vi "UHR-Fleezers Control (host) - 10.8.vi"() -> ()   [LabVIEW 2013] (continued)
        n493 = local write "Load parameters"(FALSE ("Load parameters")) -> ()
        n494 = Index Array(array="Saved AOD Raster Scan Parameter Sets", index=w859) -> (element=w858:T32)
        n495 = Unbundle By Name(w858) -> ("Scan Range AOD (nm) 2"=w857:dbl, "Step Size AOD (nm) 2"=w856:dbl, "Scan Speed AOD (nm/s) 2"=w855:dbl, "Number of scans (AOD) 2"=w854:u16)
        n496 = flat-sequence {
          tunnel: w857 -> [w865]
          tunnel: w856 -> [w864]
          tunnel: w855 -> [w863]
          tunnel: w854 -> [w866]
          frame #0 {
            n497 = local write "Scan Speed (nm/s)"(w863) -> ()
            n498 = local write "Scan Range (nm)"(w865) -> ()
            n499 = local write "Step Size (nm)"(w864) -> ()
          }
          frame #1 {
            n500 = property on="Number of F/B Scans (AOD)" class="DigNum (strict)"("Val(Sgnl)"=w866) -> ()  [unwired: 2 in, 2 out]
          }
        }
      }
      event "Trap 1 (ON/OFF)", "Trap 2 (ON/OFF)": Value Change {
        n501 = event-data() -> ()  [unwired: 7 out]
        n502 = property on="Trap 2 ON" class="Bool (strict)"("Val(Sgnl)"="Trap 2 (ON/OFF)") -> ()  [unwired: 2 in, 2 out]
        n503 = property on="Trap 1 ON" class="Bool (strict)"("Val(Sgnl)"="Trap 1 (ON/OFF)") -> ()  [unwired: 2 in, 2 out]
      }
      event "DIO count 1 (ticks)", "DIO count 2 (ticks)", "DIO count 3 (ticks)", "Interlace", "Number Interlace Sets", "Not-Interlacing Set": Value Change {
        n504 = event-data() -> ()  [unwired: 7 out]
        n505 = local read "DIO count 3 (ticks)"() -> (w879:u32)
        n506 = local read "DIO count 1 (ticks)"() -> (w881:u32)
        n507 = local read "DIO count 2 (ticks)"() -> (w880:u32)
        n508 = To Unsigned Byte Integer(number="Not-Interlacing Set") -> (unsigned 8bit integer=w870:u8)
        n509 = Add(x=w870, y=u8 1) -> (x+y=w874:u8)
        n510 = xnode "Read/Write Control"("FPGA VI Reference In"=w885, "error in"=w883, "DIO count 1 (ticks)"=w881, "DIO count 2 (ticks)"=w880, "DIO count 3 (ticks)"=w879, "Interlace ON/OFF"="Interlace", "Number Interlace Cycles"="Number Interlace Sets", "Interlace Off Parameters"=w874) -> ("error out"=w884:errorcluster)  [unwired: 1 out]
        n511 = Build Array(w881, w880, w879) -> (w872:u32[])
        n512 = Split 1D Array(array=w872, index="Number Interlace Sets") -> (first subarray=w882:u32[])  [unwired: 1 out]
        n513 = Index Array(array=w872, index=w870) -> (element=w871:u32)
        n514 = Add Array Elements(numeric array=w882) -> (sum=w876:u32)
        n515 = Select(t=w876, s="Interlace", f=w871) -> (s? t:f=→"Total Counts (ticks)":u32)
      }
      event "Reset Feedback": Value Change {
        n516 = event-data() -> ()  [unwired: 7 out]
        n517 = Unbundle By Name("Reset Feedback") -> ("Set 1"=w889:bool, "Set 2"=w888:bool)
        n518 = xnode "Read/Write Control"("FPGA VI Reference In"=w891, "error in"=w886, "FB Reset Set 1"=w889, "FB Reset Set 2"=w888) -> ("error out"=w887:errorcluster)  [unwired: 1 out]
      }
      event "PID Gains": Value Change {
        n519 = event-data() -> ()  [unwired: 7 out]
        n520 = Unbundle By Name("PID Gains") -> ("Set 1"=w895:T14, "Set 2"=w894:T14)
        n521 = xnode "Read/Write Control"("FPGA VI Reference In"=w896, "error in"=w892, "FB Gains Set 1"=w895, "FB Gains Set 2"=w894) -> ("error out"=w893:errorcluster)  [unwired: 1 out]
      }
      event "AI2 to Setpoint", "Trap Intensity\nSetpoints (V)": Value Change {
        n522 = event-data() -> ()  [unwired: 7 out]
        n523 = xnode "Read/Write Control"("FPGA VI Reference In"=w902, "error in"=w898) -> ("FPGA VI Reference Out"=w901:T19, "error out"=w900:errorcluster, "AI2 Y Sum Set 1"=w909:i16, "AI2 Y Sum Set 2"=w908:i16)
        n524 = Cluster To Array(cluster="AI2 to Setpoint") -> (array=w912:bool[])
        n525 = local read "AI2 (V)"() -> (w910:cluster{"Set 1":dbl, "Set 2":dbl})
        n526 = Or Array Elements(Boolean array=w912) -> (logical OR=w913:bool)
        n527 = Bundle By Name(cluster=w910, "Set 1"=w909, "Set 2"=w908) -> (w907:cluster{"Set 1":dbl, "Set 2":dbl})
        n528 = Divide(x=w907, y=3276.7) -> (x/y=w906:cluster{"Set 1":dbl, "Set 2":dbl})
        "AI2 (V)" <- w906
        n529 = case shown="True" w913 {
          tunnel: [w916 w933] -> w905
          tunnel: "AI2 to Setpoint" -> [_ w929]
          tunnel: "Trap Intensity\nSetpoints (V)" -> [w917 w932]
          tunnel: w906 -> [_ w926]
          frame False {
            n530 = Multiply(x=3276.7, y=w917) -> (x*y=w918:cluster{"Set 1":dbl, "Set 2":dbl})
            n531 = To Word Integer(number=w918) -> (16bit integer=w916:cluster{"Set 1":i16, "Set 2":i16})
          }
          frame True {
            n532 = Unbundle By Name(w926) -> ("Set 1"=w925:dbl, "Set 2"=w924:dbl)
            n533 = Unbundle By Name(w932) -> ("Set 1"=w931:dbl, "Set 2"=w930:dbl)
            n534 = Unbundle By Name(w929) -> ("Set 1"=w928:bool, "Set 2"=w927:bool)
            n535 = Select(t=w925, s=w928, f=w931) -> (s? t:f=w923:dbl)
            n536 = Select(t=w924, s=w927, f=w930) -> (s? t:f=w922:dbl)
            n537 = Bundle By Name(cluster=w932, "Set 1"=w923, "Set 2"=w922) -> (w920:cluster{"Set 1":dbl, "Set 2":dbl})
            n538 = local write "Trap Intensity\nSetpoints (V)"(w920) -> ()
            n539 = Multiply(x=3276.7, y=w920) -> (x*y=w921:cluster{"Set 1":dbl, "Set 2":dbl})
            n540 = To Word Integer(number=w921) -> (16bit integer=w933:cluster{"Set 1":i16, "Set 2":i16})
          }
        }
        n541 = Unbundle By Name(w905) -> ("Set 1"=w904:i16, "Set 2"=w903:i16)
        n542 = xnode "Read/Write Control"("FPGA VI Reference In"=w901, "error in"=w900, "FB Setpoint Set 1"=w904, "FB Setpoint Set 2"=w903) -> ("error out"=w899:errorcluster)  [unwired: 1 out]
      }
      event "Invert GI": Value Change {
        n543 = event-data() -> ()  [unwired: 7 out]
        n544 = xnode "Read/Write Control"("FPGA VI Reference In"=w938, "error in"=w936, "Invert GI"="Invert GI", "Invert GI 2"="Invert GI") -> ("error out"=w937:errorcluster)  [unwired: 1 out]
      }
      event "Green FB Setpoint (mV)", "Green FB Gains", "Green FB On/Off", "Current When FB OFF (%)", "Green int current ON count adj": Value Change {
        n545 = event-data() -> ()  [unwired: 7 out]
        n546 = local read "Green FB Setpoint (mV)"() -> (w945:dbl)
        n547 = local read "Current When FB OFF (%)"() -> (w948:dbl)
        n548 = Multiply(x=w945, y=3.2767) -> (x*y=w944:dbl)
        n549 = Multiply(x=w948, y=655.35) -> (x*y=w949:dbl)
        n550 = To Unsigned Word Integer(number=w949) -> (unsigned 16bit integer=w947:u16)
        n551 = local read "Green int current ON count adj"() -> (w952:u32)
        n552 = local read "Green FB Gains"() -> (w951:T14)
        n553 = local read "Green Laser ON/Interlacing"() -> (w942:bool)
        n554 = local read "Green laser mode"() -> (w941:enum32{"Laser ON", "Laser OFF", "Interlace"})
        n555 = local read "Green FB On/Off"() -> (w953:bool)
        n556 = Equal?(x=w941, y=enum32{"Laser ON", "Laser OFF", "Interlace"}."Interlace") -> (x = y?=w939:bool)
        n557 = Compound Arithmetic op=AND(w939, w953, w942) -> (w943:bool)
        n558 = xnode "Read/Write Control"("FPGA VI Reference In"=w956, "error in"=w955, "Green FB Setpoint"=w944, "Green FB On/Off"=w943, "Current Out"=w947, "Green int current ON count adj"=w952, "Green FB Gains"=w951) -> ("error out"=w954:errorcluster)  [unwired: 1 out]
      }
      event "Green laser mode", "Green Laser ON/Interlacing": Value Change {
        n559 = event-data() -> ()  [unwired: 7 out]
        n560 = case shown="True" "Green Laser ON/Interlacing" {
          tunnel: "Green laser mode" -> [_ w970]
          tunnel: [enum32{"Laser ON", "Laser OFF", "Interlace"}."Laser OFF" ("Green laser mode") w970] -> w958
          tunnel: [FALSE w966] -> w957
          frame False {
          }
          frame True {
            n561 = local read "Green FB On/Off"() -> (w967:bool)
            n562 = Equal?(x=w970, y=enum32{"Laser ON", "Laser OFF", "Interlace"}."Interlace") -> (x = y?=w968:bool)
            n563 = And(x=w968, y=w967) -> (x .and. y?=w966:bool)
          }
        }
        n564 = xnode "Read/Write Control"("FPGA VI Reference In"=w963, "error in"=w961, "Operating Mode"=w958, "Operating Mode 2"=w958, "Green FB On/Off"=w957) -> ("error out"=w962:errorcluster)  [unwired: 1 out]
      }
      event "Use mouse to move stage\n(press mouse wheel to quit)": Value Change {
        n565 = event-data() -> ()  [unwired: 7 out]
      }
      event "- phase (APD 1 Gate)", "+ phase (APD 1 Gate)": Value Change {
        n566 = event-data() -> ()  [unwired: 7 out]
        n567 = local read "Phase Adj. (APD 1 Gate)"() -> (w971:i16)
        n568 = Negate(x=w971) -> (-x=w979:i16)
        n569 = Select(t=w979, s="- phase (APD 1 Gate)", f=w971) -> (s? t:f=w978:i16)
        n570 = Or(x="- phase (APD 1 Gate)", y="+ phase (APD 1 Gate)") -> (x .or. y?=w974:bool)
        n571 = xnode "Read/Write Control"("FPGA VI Reference In"=w981, "error in"=w980, "Phase count adjustment (APD 1 Gate)"=w978) -> ("FPGA VI Reference Out"=w976:T19, "error out"=w977:errorcluster)
        n572 = xnode "Read/Write Control"("FPGA VI Reference In"=w976, "error in"=w977, "+ phase (APD 1 Gate)"=w974) -> ("error out"=w975:errorcluster)  [unwired: 1 out]
      }
      event "+ phase (APD 2 Gate)", "- phase (APD 2 Gate)": Value Change {
        n573 = event-data() -> ()  [unwired: 7 out]
        n574 = local read "Phase Adj. (APD 2 Gate)"() -> (w982:i16)
        n575 = Negate(x=w982) -> (-x=w990:i16)
        n576 = Select(t=w990, s="- phase (APD 2 Gate)", f=w982) -> (s? t:f=w989:i16)
        n577 = Or(x="- phase (APD 2 Gate)", y="+ phase (APD 2 Gate)") -> (x .or. y?=w985:bool)
        n578 = xnode "Read/Write Control"("FPGA VI Reference In"=w992, "error in"=w991, "Phase count adjustment (APD 2 Gate)"=w989) -> ("FPGA VI Reference Out"=w987:T19, "error out"=w988:errorcluster)
        n579 = xnode "Read/Write Control"("FPGA VI Reference In"=w987, "error in"=w988, "+ phase (APD 2 Gate)"=w985) -> ("error out"=w986:errorcluster)  [unwired: 1 out]
      }
      event "Phase Adj. (APD Acq)", "+ phase (APD Acq)", "- phase (APD Acq)": Value Change {
        n580 = event-data() -> ()  [unwired: 7 out]
        n581 = local read "Phase Adj. (APD Acq)"() -> (w995:i16)
        n582 = Negate(x=w995) -> (-x=w1001:i16)
        n583 = Select(t=w1001, s="+ phase (APD Acq)", f=w995) -> (s? t:f=w1000:i16)
        n584 = Or(x="+ phase (APD Acq)", y="- phase (APD Acq)") -> (x .or. y?=w996:bool)
        n585 = xnode "Read/Write Control"("FPGA VI Reference In"=w1003, "error in"=w1002, "Phase Count Adjustment (APD Acq)"=w1000) -> ("FPGA VI Reference Out"=w998:T19, "error out"=w999:errorcluster)
        n586 = xnode "Read/Write Control"("FPGA VI Reference In"=w998, "error in"=w999, "+ phase (APD Acq)"=w996) -> ("error out"=w997:errorcluster)  [unwired: 1 out]
      }
      event "Phase adj. (GI)", "+ phase (GI)", "- phase (GI)": Value Change {
        n587 = event-data() -> ()  [unwired: 7 out]
        n588 = Negate(x="Phase adj. (GI)") -> (-x=w1012:i16)
        n589 = Select(t=w1012, s="+ phase (GI)", f="Phase adj. (GI)") -> (s? t:f=w1011:i16)
        n590 = Or(x="+ phase (GI)", y="- phase (GI)") -> (x .or. y?=w1007:bool)
        n591 = xnode "Read/Write Control"("FPGA VI Reference In"=w1014, "error in"=w1013, "Phase count adjustment (GI)"=w1011) -> ("FPGA VI Reference Out"=w1009:T19, "error out"=w1010:errorcluster)
        n592 = xnode "Read/Write Control"("FPGA VI Reference In"=w1009, "error in"=w1010, "+ phase (GI)"=w1007) -> ("error out"=w1008:errorcluster)  [unwired: 1 out]
      }
      event "Phase adj. (GI) 2", "+ phase (GI) 2", "- phase (GI) 2": Value Change {
        n593 = event-data() -> ()  [unwired: 7 out]
        n594 = Negate(x="Phase adj. (GI) 2") -> (-x=w1023:i16)
        n595 = Select(t=w1023, s="+ phase (GI) 2", f="Phase adj. (GI) 2") -> (s? t:f=w1022:i16)
        n596 = Or(x="+ phase (GI) 2", y="- phase (GI) 2") -> (x .or. y?=w1018:bool)
        n597 = xnode "Read/Write Control"("FPGA VI Reference In"=w1025, "error in"=w1024, "Phase count adjustment (GI) 2"=w1022) -> ("FPGA VI Reference Out"=w1020:T19, "error out"=w1021:errorcluster)
        n598 = xnode "Read/Write Control"("FPGA VI Reference In"=w1020, "error in"=w1021, "+ phase (GI) 2"=w1018) -> ("error out"=w1019:errorcluster)  [unwired: 1 out]
      }
      event "Phase adj. (Green FB)", "- phase (Green FB)", "+ phase (Green FB)": Value Change {
        n599 = event-data() -> ()  [unwired: 7 out]
        n600 = Negate(x="Phase adj. (Green FB)") -> (-x=w1034:i16)
        n601 = Select(t=w1034, s="+ phase (Green FB)", f="Phase adj. (Green FB)") -> (s? t:f=w1033:i16)
        n602 = Or(x="+ phase (Green FB)", y="- phase (Green FB)") -> (x .or. y?=w1029:bool)
        n603 = xnode "Read/Write Control"("FPGA VI Reference In"=w1036, "error in"=w1035, "Phase count adjustment (Green FB)"=w1033) -> ("FPGA VI Reference Out"=w1031:T19, "error out"=w1032:errorcluster)
        n604 = xnode "Read/Write Control"("FPGA VI Reference In"=w1031, "error in"=w1032, "+ phase (Green FB)"=w1029) -> ("error out"=w1030:errorcluster)  [unwired: 1 out]
      }
      event "Invert APD Gate", "APD Gate ON Count", "APD Gate OFF Count", "APD Gate", "APD Integration Time (s)", "APD 1 AO Mult.", "APD 2 AO Mult.": Value Change {
        n605 = event-data() -> ()  [unwired: 7 out]
        n606 = local read "APD Integration Time (s)"() -> (w1037:dbl)
        n607 = local read "APD Gate ON Count"() -> (w1050:u32)
        n608 = local read "APD Gate OFF Count"() -> (w1049:u32)
        n609 = local read "Invert APD Gate"() -> (w1051:bool)
        n610 = local read "APD Gate"() -> (w1048:enum32{"ON", "OFF", "Interlace"})
        n611 = Multiply(x=w1037, y=40000000.0) -> (x*y=w1046:dbl)
        n612 = Reciprocal(x=w1037) -> (1/x=→"APD Acq Rate (Hz)":dbl)
        n613 = To Unsigned Long Integer(number=w1046) -> (unsigned 32bit integer=w1045:u32)
        n614 = local read "DMA Update Period (s)"() -> (w1038:dbl)
        n615 = Divide(x=w1038, y=w1037) -> (x/y=w1041:dbl)
        n616 = local read "APD 1 AO Mult."() -> (w1043:i16)
        n617 = local read "APD 2 AO Mult."() -> (w1042:i16)
        n618 = Multiply(x=2.0, y=w1041) -> (x*y=w1040:dbl)
        n619 = local write "APD Samples/FIFO Acq."(w1041) -> ()
        n620 = local write "APD Elements/DMA read"(w1040) -> ()
        n621 = xnode "Read/Write Control"("FPGA VI Reference In"=w1054, "error in"=w1053, "Invert APD Gate"=w1051, "APD Gate ON Count"=w1050, "APD Gate OFF Count"=w1049, "APD Acq Rate Count"=w1045, "APD Gate Operating Mode"=w1048, "APD 1 AO scale factor"=w1043, "APD 2 AO scale factor"=w1042) -> ("error out"=w1052:errorcluster)  [unwired: 1 out]
      }
      event "GI Frequency, ON count", "Green FB Count", "GI Frequency, OFF count": Value Change {
        n622 = event-data() -> ()  [unwired: 7 out]
        n623 = xnode "Read/Write Control"("FPGA VI Reference In"=w1060, "error in"=w1058, "Green interlace ON count"="GI Frequency, ON count", "Green interlace OFF count"="GI Frequency, OFF count", "Green interlace ON count 2"="GI Frequency, ON count", "Green interlace OFF count 2"="GI Frequency, OFF count", "Green FB Count"="Green FB Count") -> ("error out"=w1059:errorcluster)  [unwired: 1 out]
      }
      event "Number of F/B Scans (AOD)", "Scan Speed (nm/s)", "Scan BD", "Initial delta (MHz)", "Step Size (nm)", "Scan Range (nm)": Value Change {
        w1122 = 123.0  # AOM cal (nm/MHz)
        n624 = event-data() -> ()  [unwired: 7 out]
        n625 = local read "BD 1 Frequency 1 (MHz)"() -> (w1105:dbl)
        n626 = local read "AOM X Cal (nm/MHz)"() -> (w1097:dbl)
        n627 = local read "X RF Frequency Limits (MHz)"() -> (w1109:T16)
        n628 = local read "Y RF Frequency Limits (MHz)"() -> (w1106:T16)
        n629 = local read "BD 2 Frequency 1 (MHz)"() -> (w1111:dbl)
        n630 = Negate(x="Scan Range (nm)") -> (-x=w1075:dbl)
        n631 = Divide(x=w1075, y=w1097) -> (x/y=w1079:dbl)
        n632 = Select(t=w1109, s="Scan BD", f=w1106) -> (s? t:f=w1108:T16)
        n633 = Select(t=w1105, s="Scan BD", f=w1111) -> (s? t:f=w1110:dbl)
        n634 = Unbundle By Name(w1108) -> ("Maximum"=w1117:dbl, "Minimum"=w1116:dbl)
        n635 = Add(x=w1079, y=w1110) -> (x+y=w1114:dbl)
        n636 = Divide(x=w1075, y="Step Size (nm)") -> (x/y=w1094:dbl)
        n637 = Divide(x="Step Size (nm)", y=w1097) -> (x/y=w1103:dbl)
        n638 = Absolute Value(x=w1094) -> (abs(x)=w1078:dbl)
        n639 = Sign(1:w1075) -> (0:w1076:dbl)
        n640 = In Range and Coerce(upper limit=w1117, x=w1114, lower limit=w1116) -> (coerced(x)=w1113:dbl, In Range?=w1115:bool)
        n641 = To Unsigned Quad Integer(1:w1078) -> (0:w1093:u64)
        "Scan steps (AOD)" <- w1093
        n642 = call "IR AOM freq to word.vi"("Frequency In (MHz)"=w1103) -> ("Frequency Word Out (double)"=w1100:dbl)
        n643 = Multiply(x=w1076, y=w1100) -> (x*y=w1077:dbl)
        n644 = Subtract(x=w1114, y=w1113) -> (x-y=w1112:dbl)
        n645 = To Quad Integer(1:w1077) -> (0:w1099:i64)
        "Incr. int (AOD)" <- w1099
        n646 = Subtract(x=w1079, y=w1112) -> (x-y=w1098:dbl)
        "Scan Range (MHz)" <- w1098
        n647 = Select(t=w1079, s=w1115, f=w1098) -> (s? t:f=w1118:dbl)
        n648 = Multiply(x=w1098, y=w1097) -> (x*y=w1096:dbl)
        n649 = Decrement(x=w1093) -> (x-1=w1146:u64)
        n650 = Negate(x=w1096) -> (-x=w1092:dbl)
        n651 = local write "Scan Range (nm)"(w1092) -> ()
        n652 = Divide(x=w1118, y=w1146) -> (x/y=w1102:dbl)
        "Scan Increment (MHz)" <- w1102
        n653 = call "IR AOM freq to word.vi"("Frequency In (MHz)"=w1102) -> ("Frequency Word Out (double)"=w1101:dbl)
        n654 = Divide(x="Step Size (nm)", y="Scan Speed (nm/s)") -> (x/y=w1089:dbl)
        n655 = To Quad Integer(1:w1101) -> ()  [unwired: 1 out]
        n656 = local read "Number Interlace Sets"() -> (w1073:u8)
        n657 = local read "AI Count (ticks)"() -> (w1074:u32)
        n658 = local read "Total Counts (ticks)"() -> (w1072:u32)
        n659 = local read "# Samples/trap"() -> (w1104:u32)
        n660 = Multiply(x=w1074, y=w1073) -> (x*y=w1071:u32)
        n661 = Divide(x=w1072, y=w1071) -> (x/y=w1070:dbl)
        n662 = Select(t=w1105, s="Scan BD", f=w1111) -> (s? t:f=w1143:dbl)
        "Initial freq. (MHz)" <- w1143
        n663 = Add(x=w1118, y=w1143) -> (x+y=→"Final freq. (MHz)":dbl)
        n664 = Divide(x=w1072, y=40000000.0) -> (x/y=w1088:dbl)
        n665 = Divide(x=w1089, y=w1088) -> (x/y=w1087:dbl)
        n666 = To Unsigned Quad Integer(1:w1087) -> (0:w1062:u64)
        n667 = Quotient & Remainder(x=w1062, y=u64 2) -> (x-y*floor(x/y)=w1066:u64)  [unwired: 1 out]
        n668 = Equal?(x=w1066, y=u64 0) -> (x = y?=w1064:bool)
        n669 = Decrement(x=w1062) -> (x-1=w1063:u64)
        n670 = Select(t=w1062, s=w1064, f=w1063) -> (s? t:f=w1061:u64)
        "Cycles/step (AOD)" <- w1061
        n671 = xnode "Read/Write Control"("FPGA VI Reference In"=w1154, "error in"=w1153, "Scan steps"=w1093, "Number of scans"="Number of F/B Scans (AOD)", "Cycles per step"=w1061, "Scan freq.  increment"=w1099, "Scan BD"="Scan BD") -> ("error out"=w1152:errorcluster)  [unwired: 1 out]
        n672 = Multiply(x=w1093, y=w1061) -> (x*y=w1147:u64)
        n673 = Multiply(x=w1147, y=u64 2) -> (x*y=w1069:u64)
        n674 = Multiply(x=w1070, y=w1069) -> (x*y=w1068:dbl)
        "Data points/scan (f/b)" <- w1068
        n675 = Multiply(x=w1068, y="Number of F/B Scans (AOD)") -> (x*y=w1150:dbl)
        "Data points/scans" <- w1150
        n676 = Divide(x=w1150, y=w1104) -> (x/y=→"N sets should be saved":dbl)
        n677 = Multiply(x=w1147, y=w1088) -> (x*y=w1086:dbl)
        "Time/Scan (s) (AOD)" <- w1086
        n678 = Select(t=w1118, s="Scan BD", f=0.0) -> (s? t:f=w1144:dbl)
        n679 = Select(t=0.0, s="Scan BD", f=w1118) -> (s? t:f=w1140:dbl)
        n680 = local read "BD 2 Frequency 2 (MHz)"() -> (w1136:dbl)
        n681 = local read "BD 1 Frequency 2 (MHz)"() -> (w1139:dbl)
        n682 = Add(x=w1140, y=w1111) -> (x+y=w1137:dbl)
        n683 = Add(x=w1105, y=w1144) -> (x+y=w1138:dbl)
        n684 = Multiply(x=w1086, y=2.0) -> (x*y=w1085:dbl)
        n685 = Multiply(x=w1085, y="Number of F/B Scans (AOD)") -> (x*y=w1082:dbl)
        n686 = Divide(x=w1082, y=60.0) -> (x/y=→"Time to Finish All (min)":dbl)
        n687 = Add(x="Trap 2 Bead Size (nm)", y="Trap 1 Bead Size (nm)") -> (x+y=w1126:dbl)
        n688 = local read "Initial delta (MHz)"() -> (w1123:dbl)
        n689 = Divide(x=w1126, y=2.0) -> (x/y=w1120:dbl)
        n690 = Subtract(x=w1137, y=w1136) -> (x-y=w1134:dbl)
        n691 = Subtract(x=w1138, y=w1139) -> (x-y=w1135:dbl)
        n692 = Square(x=w1134) -> (x^2=w1133:dbl)
        n693 = Square(x=w1135) -> (x^2=w1132:dbl)
        n694 = Add(x=w1132, y=w1133) -> (x+y=w1131:dbl)
        n695 = Square Root(x=w1131) -> (sqrt(x)=w1130:dbl)
        "Final delta (MHz)" <- w1130
        n696 = Multiply(x=w1122, y=w1130) -> (x*y=w1129:dbl)
        n697 = Multiply(x=w1123, y=w1122) -> (x*y=w1121:dbl)
        n698 = Subtract(x=w1121, y=w1120) -> (x-y=→"Initial sep (nm)":dbl)
        n699 = Subtract(x=w1129, y=w1120) -> (x-y=→"Final sep (nm)":dbl)
      }
      event "Raster Scanning...": Value Change {
        n700 = event-data() -> ("NewVal"=w1155:bool)  [unwired: 6 out]
        n701 = case shown="True" w1155 {
          frame False {
          }
          frame True {
            n702 = property on="BD 1 Frequency 1 (MHz)" class="DigNum (strict)"("Val(Sgnl)"=65.0 ("Value (Signaling)")) -> ()  [unwired: 2 in, 2 out]
          }
        }
      }
      event "Freq or Amp switch first", "Swap F1 and F2", "Freq switch delay", "Amp switch delay": Value Change {
        n703 = event-data() -> ()  [unwired: 7 out]
        n704 = local read "Freq or Amp switch first"() -> (w1157:bool)
        n705 = local read "Amp switch delay"() -> (w1158:u16)
        n706 = local read "Freq switch delay"() -> (w1160:u16)
        n707 = local read "Swap F1 and F2"() -> (w1159:bool)
        n708 = xnode "Read/Write Control"("FPGA VI Reference In"=w1163, "error in"=w1162, "Freq switch delay"=w1160, "Swap F1 and F2"=w1159, "Amp switch delay"=w1158, "Freq or Amp switch first"=w1157) -> ("error out"=w1161:errorcluster)  [unwired: 1 out]
      }
      event "Scan steps (MCL)", "Number of scans (MCL)", "Scan Range (V)\n(of steps)", "2D or 1D Scan", "N APD Samp/step", "Fast Scan Dir", "Continuous MCL Scanning", "Scan lines (y)": Value Change {
        w1165 = 32767.0 ("y")
        n709 = event-data() -> ()  [unwired: 7 out]
        n710 = Select(t="Scan lines (y)", s="2D or 1D Scan", f="Number of scans (MCL)") -> (s? t:f=w1170:u64)
        n711 = Decrement(x="Scan steps (MCL)") -> (x-1=w1186:u64)
        n712 = Divide(x="Scan Range (V)\n(of steps)", y=w1186) -> (x/y=w1185:dbl)
        "Desired Scan Incr (V)" <- w1185
        n713 = local read "APD Integration Time (s)"() -> (w1178:dbl)
        n714 = Multiply(x=w1185, y=w1165) -> (x*y=w1194:dbl)
        n715 = Divide(x=w1194, y=10.0) -> (x/y=w1184:dbl)
        "Desired incr (int)" <- w1184
        n716 = local read "Update Count (MCL)"() -> (w1190:u32)
        n717 = Round Toward -Infinity(1:w1184) -> (0:w1193:dbl)
        n718 = To Word Integer(number=w1193) -> (16bit integer=w1168:i16)
        "Actual Incr. int (MCL)" <- w1168
        n719 = Multiply(x=w1178, y=40000000.0) -> (x*y=w1191:dbl)
        n720 = Divide(x=w1191, y=w1190) -> (x/y=w1189:dbl)
        n721 = Multiply(x=i16 10, y=w1168) -> (x*y=w1166:i16)
        n722 = Multiply(x="N APD Samp/step", y=w1189) -> (x*y=w1188:dbl)
        "Cycles/step (MCL)" <- w1188
        n723 = Divide(x=w1166, y=w1165) -> (x/y=→"Actual MCL Inc (V)":dbl)
        n724 = Multiply(x="N APD Samp/step", y="Scan steps (MCL)") -> (x*y=w1180:dbl)
        n725 = local read "APD Samples/FIFO Acq."() -> (w1177:dbl)
        n726 = Multiply(x=w1180, y=u64 2) -> (x*y=w1179:dbl)
        "Data points/scan (f+b)" <- w1179
        n727 = Multiply(x=w1179, y=w1170) -> (x*y=w1197:dbl)
        "Data points/scans (MCL)" <- w1197
        n728 = Multiply(x=w1178, y=w1179) -> (x*y=w1171:dbl)
        "Time/f+b scan (s) (MCL)" <- w1171
        n729 = Divide(x=w1197, y=w1177) -> (x/y=→"N sets should be saved (MCL)":dbl)
        n730 = Multiply(x=w1171, y=w1170) -> (x*y=→"Total Time (s)":dbl)
        n731 = Not(x="Fast Scan Dir") -> (.not. x?=w1175:bool)
        n732 = xnode "Read/Write Control"("FPGA VI Reference In"=w1201, "error in"=w1200, "Scan steps (MCL)"="Scan steps (MCL)", "Number of scans (MCL)"=w1170, "Cycles per step (MCL)"=w1188, "Scan freq.  increment (MCL)"=w1168, "1D or 2D Scan?"="2D or 1D Scan", "MCL Scan Axis"=w1175, "Cont. Scan (MCL)"="Continuous MCL Scanning") -> ("error out"=w1199:errorcluster)  [unwired: 1 out]
      }
      event Key Down {
        n733 = event-data() -> ("VKey"=w1203:T33)  [unwired: 10 out]
        n734 = local read "z nudge increment (um)"() -> (w1202:dbl)
        n735 = case shown="\"F11\"" w1203 {
          tunnel: "lateral step size (mm)" -> [w1206 w1211 w1216 w1224 _ _ _ _ _ _ _ _ _ _ _ _ _ _ _ _ _ _ _ _ _ _ _ _ _ _ _ _ _ _ _ _ _ _ _ _ _ _ _ _ _ _ _ _ _ _ _ _ _ _ _ _]
          tunnel: w1202 -> [_ _ _ _ w1227 w1234 _ _ _ _ _ _ _ _ _ _ _ _ _ _ _ _ _ _ _ _ _ _ _ _ _ _ _ _ _ _ _ _ _ _ _ _ _ _ _ _ _ _ _ _ _ _ _ _ _ _]
          frame "Up" {
            w1208 = 0.0 ("element")
            n736 = Negate(x=w1206) -> (-x=w1205:dbl)
            n737 = Build Array(w1208, w1205, w1208) -> (w1207:dbl[])
            n738 = call "CONEX_FUNCTIONAL_GLOBAL.vi"("Axis"=enum16{"X", "Y", "Z", "XY", "XZ", "YZ", "XYZ"}."Y", "Position"=w1207, "Command"=T20."REL MOVE") -> ()  [unwired: 6 in, 3 out]
          }
          frame "Down" {
            w1213 = 0.0 ("element")
            n739 = Build Array(w1213, w1211, w1213) -> (w1212:dbl[])
            n740 = call "CONEX_FUNCTIONAL_GLOBAL.vi"("Axis"=enum16{"X", "Y", "Z", "XY", "XZ", "YZ", "XYZ"}."Y", "Position"=w1212, "Command"=T20."REL MOVE") -> ()  [unwired: 6 in, 3 out]
          }
          frame "Left" {
            w1217 = 0.0 ("element")
            n741 = Build Array(w1216, w1217, w1217) -> (w1218:dbl[])
            n742 = call "CONEX_FUNCTIONAL_GLOBAL.vi"("Axis"=enum16{"X", "Y", "Z", "XY", "XZ", "YZ", "XYZ"}."X", "Position"=w1218, "Command"=T20."REL MOVE") -> ()  [unwired: 6 in, 3 out]
          }
          frame "Right" {
            w1222 = 0.0 ("element")
            n743 = Negate(x=w1224) -> (-x=w1223:dbl)
            n744 = Build Array(w1223, w1222, w1222) -> (w1221:dbl[])
            n745 = call "CONEX_FUNCTIONAL_GLOBAL.vi"("Axis"=enum16{"X", "Y", "Z", "XY", "XZ", "YZ", "XYZ"}."X", "Position"=w1221, "Command"=T20."REL MOVE") -> ()  [unwired: 6 in, 3 out]
          }
          frame "PageUp" {
            w1231 = 0.0 ("element")
            n746 = Divide(x=w1227, y=1000.0) -> (x/y=w1229:dbl)
            n747 = Build Array(w1231, w1231, w1229) -> (w1230:dbl[])
            n748 = call "CONEX_FUNCTIONAL_GLOBAL.vi"("Axis"=enum16{"X", "Y", "Z", "XY", "XZ", "YZ", "XYZ"}."Z", "Position"=w1230, "Command"=T20."REL MOVE") -> ()  [unwired: 6 in, 3 out]
          }
          frame "PageDown" {
            w1238 = 0.0 ("element")
            n749 = Divide(x=w1234, y=-1000.0) -> (x/y=w1236:dbl)
            n750 = Build Array(w1238, w1238, w1236) -> (w1237:dbl[])
            n751 = call "CONEX_FUNCTIONAL_GLOBAL.vi"("Axis"=enum16{"X", "Y", "Z", "XY", "XZ", "YZ", "XYZ"}."Z", "Position"=w1237, "Command"=T20."REL MOVE") -> ()  [unwired: 6 in, 3 out]
          }
          frame Default {
          }
          frame "Insert" {
          }
          frame "Delete" {
          }
          frame "Home" {
          }
          frame "End" {
          }
          frame "Escape" {
          }
          frame "Help" {
          }
          frame "Pause" {
          }
          frame "ScrollLock" {
          }
          frame "F1" {
          }
          frame "F2" {
          }
          frame "F3" {
          }
          frame "F4" {
          }
          frame "F5" {
          }
          frame "F6" {
          }
          frame "F7" {
          }
          frame "F8" {
          }
          frame "F9" {
            n752 = local read "Trap 1 (ON/OFF)"() -> (w1242:bool)
            n753 = Not(x=w1242) -> (.not. x?=w1241:bool)
            n754 = property on="Trap 1 (ON/OFF)" class="Bool (strict)"("Val(Sgnl)"=w1241) -> ()  [unwired: 2 in, 2 out]
          }
          frame "F10" {
            n755 = local read "Trap 2 (ON/OFF)"() -> (w1244:bool)
            n756 = Not(x=w1244) -> (.not. x?=w1243:bool)
            n757 = property on="Trap 2 (ON/OFF)" class="Bool (strict)"("Val(Sgnl)"=w1243) -> ()  [unwired: 2 in, 2 out]
          }
          frame "F11" {
            n758 = local read "Sample Channel Flow"() -> (w1247:bool)
            n759 = Not(x=w1247) -> (.not. x?=w1246:bool)
            n760 = property on="Sample Channel Flow" class="Bool (strict)"("Val(Sgnl)"=w1246) -> ()  [unwired: 2 in, 2 out]
            n761 = Wait (ms)(milliseconds to wait=u32 1500) -> ()  [unwired: 1 out]
          }
          frame "F12" {
            n762 = local read "Use mouse to move stage\n(press mouse wheel to quit)"() -> (w1249:bool)
            n763 = Not(x=w1249) -> (.not. x?=w1248:bool)
            n764 = case shown="False" w1248 {
              frame False {
                n765 = flat-sequence {
                  frame #0 {
                    n766 = dll-call lib="user32.dll" fn="ShowCursor" label="Call Library Function"("Enable"=1) -> ()  [unwired: 3 in, 4 out]
                  }
                  frame #1 {
                    n767 = Wait (ms)(milliseconds to wait=u32 1000) -> ()  [unwired: 1 out]
                  }
                }
                n768 = property class="VI"() -> ("Panel"=w1251:refnum<vi>)  [unwired: 2 in, 2 out]
                n769 = property class="Pnl"(reference=w1251) -> ("Panes[]"=w1252:refnum<vi>[])  [unwired: 1 in, 2 out]
                n770 = for {
                  tunnel: w1252 -> [w1256] mode=indexing
                  tunnel: T30."Always On" ("Horizontal Scrollbar Visibility") -> [w1257]
                  n771 = property class="Pane"(reference=w1256, "HorizScrollbarVisibility"=w1257) -> (reference out=w1255:refnum<vi>)  [unwired: 1 in, 1 out]
                  n772 = property class="Pane"(reference=w1255, "VertScrollbarVisibility"=w1257) -> ()  [unwired: 1 in, 2 out]
                }
              }
              frame True {
                n773 = property class="VI"() -> ("Panel"=w1259:refnum<vi>)  [unwired: 2 in, 2 out]
                n774 = property class="Pnl"(reference=w1259) -> ("Panes[]"=w1260:refnum<vi>[])  [unwired: 1 in, 2 out]
                n775 = flat-sequence {
                  frame #0 {
                    n776 = dll-call lib="user32.dll" fn="ShowCursor" label="Call Library Function"("Enable"=0) -> ()  [unwired: 3 in, 4 out]
                  }
                  frame #1 {
                    n777 = Wait (ms)(milliseconds to wait=u32 1000) -> ()  [unwired: 1 out]
                  }
                }
                n778 = for {
                  tunnel: w1260 -> [w1265] mode=indexing
                  tunnel: T30."Always Off" ("Horizontal Scrollbar Visibility") -> [w1263]
                  n779 = property class="Pane"(reference=w1265, "HorizScrollbarVisibility"=w1263) -> (reference out=w1264:refnum<vi>)  [unwired: 1 in, 1 out]
                  n780 = property class="Pane"(reference=w1264, "VertScrollbarVisibility"=w1263) -> ()  [unwired: 1 in, 2 out]
                }
              }
            }
            n781 = local write "Use mouse to move stage\n(press mouse wheel to quit)"(w1248) -> ()
          }
          frame "F13" {
          }
          frame "F14" {
          }
          frame "F15" {
          }
          frame "F16" {
          }
          frame "F17" {
          }
          frame "F18" {
          }
          frame "F19" {
          }
          frame "F20" {
          }
          frame "F21" {
          }
          frame "F22" {
          }
          frame "F23" {
          }
          frame "F24" {
          }
          frame "Play" {
          }
          frame "VolumeUp" {
          }
          frame "VolumeDown" {
          }
          frame "Mute" {
          }
          frame "Two Byte Char" {
          }
          frame "Break" {
          }
          frame "Clear" {
          }
          frame "NumLock" {
          }
          frame "Caps" {
          }
          frame "Opt" {
          }
          frame "Cmd" {
          }
          frame "Alt" {
          }
          frame "Ctrl" {
          }
          frame "Shift" {
          }
          frame "Return" {
          }
          frame "Enter" {
          }
          frame "ASCII" {
          }
        }
      }
      event "Read Cal": Value Change {
        w1267 = 1000.0 ("y")
        n782 = event-data() -> ()  [unwired: 7 out]
        n783 = local read "Save file name"() -> (w1292:path)
        n784 = local write "Read Cal"(FALSE ("Read Cal")) -> ()
        n785 = Strip Path(path=w1292) -> (stripped path=w1291:path)  [unwired: 1 out]
        n786 = Path To String(path=w1291) -> (string=w1290:string)
        n787 = Concatenate Strings(w1290, "\\current.cal" ("string")) -> (w1288:string)
        n788 = String To Path(string=w1288) -> (path=w1287:path)
        n789 = Open/Create/Replace File(file path (use dialog)=w1287, operation (0:open)=T23."open", access (0:read/write)=enum16{"read/write", "read-only", "write-only"}."read-only") -> (refnum out=w1295:refnum<file>, error out=w1281:errorcluster)  [unwired: 1 in, 3 out]
        n790 = Deny Access(4:w1281, 7:w1295) -> (0:w1280:errorcluster, 3:w1286:refnum<file>)  [unwired: 1 out]
        n791 = Read from Binary File(5:0.0, 8:w1280, 9:T31."big-endian, network order" ("byte order (0:big-endian, network order)"), 10:-1 ("count (1)"), 11:w1286) -> (0:w1279:errorcluster, 2:w1277:dbl[], 3:w1282:refnum<file>)  [unwired: 2 out]
        n792 = Array To Cluster(array=w1277) -> (cluster=w1276:T34)
        n793 = Unbundle(w1276) -> ("[0]"=w1275:dbl, "[1]"=w1274:dbl, "[2]"=w1273:dbl, "[3]"=w1272:dbl, "[4]"=w1271:dbl, "[5]"=w1270:dbl)
        n794 = Close File(refnum=w1282, error in=w1279) -> (error out=→"Read cal error":errorcluster)  [unwired: 1 out]
        n795 = Multiply(x=w1270, y=w1267) -> (x*y=w1268:dbl)
        n796 = local write "T2 kappa_x (pN/nm)"(w1272) -> ()
        n797 = local write "T1 kappa_x (pN/nm)"(w1273) -> ()
        n798 = local write "T1 alpha_x (nm/V)"(w1275) -> ()
        n799 = local write "T2 alpha_x (nm/V)"(w1274) -> ()
        n800 = Multiply(x=w1271, y=w1267) -> (x*y=w1269:dbl)
        n801 = local write "T1 offset_x (mV)"(w1269) -> ()
        n802 = local write "T2 offset_x (mV)"(w1268) -> ()
      }
      event "Abort MCL Scan": Value Change {
        n803 = event-data() -> ()  [unwired: 7 out]
        n804 = local write "MCL Scanning"(FALSE ("MCL Scanning")) -> ()
        n805 = xnode "Read/Write Control"("FPGA VI Reference In"=w1300, "error in"=w1299, "Abort scan (MCL)"="Abort MCL Scan") -> ("error out"=w1298:errorcluster)  [unwired: 1 out]
      }
      event "Update Count (MCL)": Value Change {
        n806 = event-data() -> ()  [unwired: 7 out]
        n807 = xnode "Read/Write Control"("FPGA VI Reference In"=w1304, "error in"=w1303, "MCL count"="Update Count (MCL)") -> ("error out"=w1302:errorcluster)  [unwired: 1 out]
      }
      event "Phase adjust (MCL)", "+ phase (MCL)", "- phase (MCL)": Value Change {
        n808 = event-data() -> ()  [unwired: 7 out]
        n809 = Negate(x="Phase adjust (MCL)") -> (-x=w1313:i16)
        n810 = Select(t=w1313, s="- phase (MCL)", f="Phase adjust (MCL)") -> (s? t:f=w1311:i16)
        n811 = Or(x="- phase (MCL)", y="+ phase (MCL)") -> (x .or. y?=w1306:bool)
        n812 = xnode "Read/Write Control"("FPGA VI Reference In"=w1315, "error in"=w1314, "Phase count adjustment (MCL)"=w1311) -> ("FPGA VI Reference Out"=w1307:T19, "error out"=w1308:errorcluster)
        n813 = xnode "Read/Write Control"("FPGA VI Reference In"=w1307, "error in"=w1308, "+ phase (MCL)"=w1306) -> ("error out"=w1305:errorcluster)  [unwired: 1 out]
      }
      event "Abort AOD Scan": Value Change {
        n814 = event-data() -> ()  [unwired: 7 out]
        n815 = xnode "Read/Write Control"("FPGA VI Reference In"=w1319, "error in"=w1318, "Abort scan"="Abort AOD Scan") -> ("error out"=w1317:errorcluster)  [unwired: 1 out]
      }
      event "Continuous AOD Scanning": Value Change {
        n816 = event-data() -> ()  [unwired: 7 out]
        n817 = xnode "Read/Write Control"("FPGA VI Reference In"=w1323, "error in"=w1322, "Cont. Scan"="Continuous AOD Scanning") -> ("error out"=w1321:errorcluster)  [unwired: 1 out]
      }
      event "Index": Value Change {
        n818 = event-data() -> ()  [unwired: 7 out]
        n819 = call "Create new save file.vi"("Insert"="", "Ext"=".dat" ("string"), "Index In"="Index") -> ("Path Out"=→"Save file name":path, "Index Out"=w1324:dbl)
        "Save index" <- w1324
        n820 = local write "Index"(w1324) -> ()
      }
      event "AO1", "AO2": Value Change {
        w1339 = 10.0 ("y")
        w1338 = 32767.0 ("y")
        n821 = event-data() -> ()  [unwired: 7 out]
        n822 = local read "AO2"() -> (w1337:dbl)
        n823 = local read "AO1"() -> (w1334:dbl)
        n824 = Multiply(x=w1334, y=w1338) -> (x*y=w1333:dbl)
        n825 = Multiply(x=w1337, y=w1338) -> (x*y=w1336:dbl)
        n826 = Divide(x=w1333, y=w1339) -> (x/y=w1332:dbl)
        n827 = Divide(x=w1336, y=w1339) -> (x/y=w1335:dbl)
        n828 = To Word Integer(number=w1332) -> (16bit integer=w1340:i16)
        n829 = To Word Integer(number=w1335) -> (16bit integer=w1341:i16)
        n830 = xnode "Read/Write Control"("FPGA VI Reference In"=w1331, "error in"=w1330, "AO1"=w1340, "AO2"=w1341) -> ("error out"=w1329:errorcluster)  [unwired: 1 out]
      }
      event "Inject Bottom": Value Change {
        n831 = event-data() -> ()  [unwired: 7 out]
        n832 = disable-structure shown="Enabled" {
          disable-tunnel: "Inject Bottom" -> [w1343 w1383]
          frame Disabled {
            n833 = local read "Chemyx Syringe Pump Serial Port"() -> (w1344:refnum<visa-resource-name>)
            n834 = local read "Pump write delay (ms)"() -> (w1345:dbl)
            n835 = case shown="True" w1343 {
              tunnel: w1345 -> [w1351 w1365]
              tunnel: w1344 -> [w1348 w1364]
              frame False {
                n836 = flat-sequence {
                  tunnel: w1348 -> [w1352]
                  tunnel: [w1352] -> w1349
                  tunnel: w1351 -> [_]
                  tunnel: [w1355] -> w1350
                  tunnel: w1349 -> [w1355]
                  tunnel: w1350 -> [w1356]
                  tunnel: [w1356] -> w1346
                  tunnel: [w1358] -> w1347
                  tunnel: w1346 -> [w1358]
                  tunnel: w1347 -> [w1360]
                  frame #0 {
                    n837 = call "Write to pump.vi"("string"="enter pump1", "VISA resource name"=w1352) -> ()  [unwired: 1 out]
                  }
                  frame #1 {
                    n838 = Wait (ms)(milliseconds to wait="Pump pause delay (ms)") -> ()  [unwired: 1 out]
                  }
                  frame #2 {
                    n839 = call "Write to pump.vi"("string"="stop", "VISA resource name"=w1356) -> ()  [unwired: 1 out]
                  }
                  frame #3 {
                    n840 = Wait (ms)(milliseconds to wait=u32 500) -> ()  [unwired: 1 out]
                  }
                  frame #4 {
                    n841 = call "Write to pump.vi"("string"="stop", "VISA resource name"=w1360) -> ()  [unwired: 1 out]
                  }
                }
              }
              frame True {
                n842 = flat-sequence {
                  tunnel: w1364 -> [w1374]
                  tunnel: w1365 -> [w1369]
                  tunnel: w1365 -> [w1376]
                  tunnel: w1364 -> [w1377]
                  tunnel: [w1377] -> w1362
                  tunnel: [w1379] -> w1363
                  tunnel: w1362 -> [w1379]
                  tunnel: w1363 -> [w1381]
                  frame #0 {
                    n843 = local read "All Pump Parameters"() -> (w1368:T5)
                    n844 = Unbundle By Name(w1368) -> ("Pump 1"=w1375:T35)
                    n845 = call "Set pump parameters.vi"("Pump write delay (ms)"=w1369, "Volume (uL)"="Ch 2 Inject Volume (uL)", "Rate (uL/h)"="Ch 1 Inject Rate (ul/h)", "Units"=4.0, "Pump #"=1.0, "Pump Parameters In"=w1375, "VISA resource name"=w1374) -> ("Pump Parameters Out"=w1367:T35)  [unwired: 3 in]
                    n846 = Bundle By Name(cluster=w1368, "Pump 1"=w1367) -> (w1366:T5)
                    n847 = local write "All Pump Parameters"(w1366) -> ()
                  }
                  frame #1 {
                    n848 = Wait (ms)(milliseconds to wait=w1376) -> ()  [unwired: 1 out]
                  }
                  frame #2 {
                    n849 = call "Write to pump.vi"("string"="start", "VISA resource name"=w1377) -> ()  [unwired: 1 out]
                  }
                  frame #3 {
                    n850 = Wait (ms)(milliseconds to wait=u32 500) -> ()  [unwired: 1 out]
                  }
                  frame #4 {
                    n851 = call "Write to pump.vi"("string"="start", "VISA resource name"=w1381) -> ()  [unwired: 1 out]
                  }
                }
              }
            }
          }
          frame Enabled {
            n852 = call "hamilton_controller.vi"("Open?"=w1383, "valve"=enum16{"A", "B", "C", "D", "ALL"}."B", "action"=T21."MOVE VALVE") -> ()  [unwired: 8 in, 1 out]
          }
        }
      }
      event "Inject Top": Value Change {
        n853 = event-data() -> ()  [unwired: 7 out]
        n854 = disable-structure shown="Enabled" {
          disable-tunnel: "Inject Top" -> [_ w1427]
          frame Disabled {
            n855 = local read "Pump write delay (ms)"() -> (w1388:dbl)
            n856 = case shown="False" w1389 {
              tunnel: w1388 -> [w1395 w1409]
              tunnel: "Chemyx Syringe Pump Serial Port" -> [w1392 w1408]
              frame False {
                n857 = flat-sequence {
                  tunnel: w1392 -> [w1396]
                  tunnel: [w1396] -> w1393
                  tunnel: w1395 -> [_]
                  tunnel: [w1399] -> w1394
                  tunnel: w1393 -> [w1399]
                  tunnel: w1394 -> [w1400]
                  tunnel: [w1400] -> w1390
                  tunnel: [w1402] -> w1391
                  tunnel: w1390 -> [w1402]
                  tunnel: w1391 -> [w1404]
                  frame #0 {
                    n858 = call "Write to pump.vi"("string"="enter pump3", "VISA resource name"=w1396) -> ()  [unwired: 1 out]
                  }
                  frame #1 {
                    n859 = local read "Pump pause delay (ms)"() -> (w1398:u32)
                    n860 = Wait (ms)(milliseconds to wait=w1398) -> ()  [unwired: 1 out]
                  }
                  frame #2 {
                    n861 = call "Write to pump.vi"("string"="stop", "VISA resource name"=w1400) -> ()  [unwired: 1 out]
                  }
                  frame #3 {
                    n862 = Wait (ms)(milliseconds to wait=u32 0) -> ()  [unwired: 1 out]
                  }
                  frame #4 {
                    n863 = call "Write to pump.vi"("string"="stop", "VISA resource name"=w1404) -> ()  [unwired: 1 out]
                  }
                }
              }
              frame True {
                n864 = flat-sequence {
                  tunnel: w1408 -> [w1418]
                  tunnel: w1409 -> [w1413]
                  tunnel: w1409 -> [w1420]
                  tunnel: w1408 -> [w1421]
                  tunnel: [w1421] -> w1406
                  tunnel: [w1424] -> w1407
                  tunnel: w1406 -> [w1424]
                  tunnel: w1407 -> [w1425]
                  frame #0 {
                    n865 = local read "All Pump Parameters"() -> (w1412:T5)
                    n866 = Unbundle By Name(w1412) -> ("Pump 3"=w1419:T35)
                    n867 = call "Set pump parameters.vi"("Pump write delay (ms)"=w1413, "Volume (uL)"="Ch 3 Inject Volume (uL)", "Rate (uL/h)"="Ch 3 Inject Rate (ul/h)", "Units"=4.0, "Pump #"=3.0, "Pump Parameters In"=w1419, "VISA resource name"=w1418) -> ("Pump Parameters Out"=w1411:T35)  [unwired: 3 in]
                    n868 = Bundle By Name(cluster=w1412, "Pump 3"=w1411) -> (w1410:T5)
                    n869 = local write "All Pump Parameters"(w1410) -> ()
                  }
                  frame #1 {
                    n870 = Wait (ms)(milliseconds to wait=w1420) -> ()  [unwired: 1 out]
                  }
                  frame #2 {
                    n871 = call "Write to pump.vi"("string"="start", "VISA resource name"=w1421) -> ()  [unwired: 1 out]
                  }
                  frame #3 {
                    n872 = Wait (ms)(milliseconds to wait=u32 500) -> ()  [unwired: 1 out]
                  }
                  frame #4 {
                    n873 = call "Write to pump.vi"("string"="start", "VISA resource name"=w1425) -> ()  [unwired: 1 out]
                  }
                }
              }
            }
          }
          frame Enabled {
            n874 = call "hamilton_controller.vi"("Open?"=w1427, "valve"=enum16{"A", "B", "C", "D", "ALL"}."A", "action"=T21."MOVE VALVE") -> ()  [unwired: 8 in, 1 out]
          }
        }
      }
      event "Inject Valve B": Value Change {
        n875 = event-data() -> ()  [unwired: 7 out]
        n876 = disable-structure shown="Enabled" {
          disable-tunnel: "Inject Valve B" -> [w1431 w1451]
          frame Disabled {
